vi "Create UA Client.vi"(8 "error in (no error)":errorcluster, 11 "OPCUA Setting In":T3) -> (0 "error out":errorcluster, 1 "Connected?":bool, 2 "NodeID Out":string, 3 "OPC UA client refnum out":T2)   [LabVIEW 2024, in "OPCUA.lvlib"]
uses:
  OPCUA.lvlib
  OPCUA Setting.ctl
  <vilib>/OPCUA/controls/OPC UA Client Refnum.ctl
  <vilib>/OPCUA/NI OPC UA Client.lvlib
panel:
  in  "security policy":T1
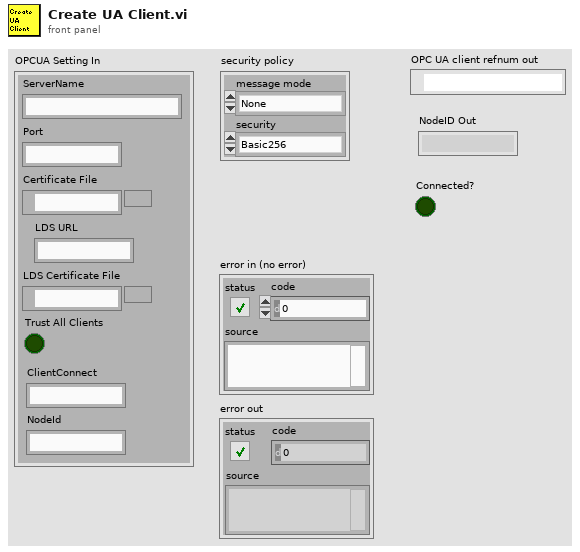
[diagram p1: front panel]
types:
  T1 = cluster{"message mode":enum16{"None", "Sign", "Sign and Encrypt"}, "security":enum16{"Basic256", "Basic128Rsa15"}}
  T2 = typedef "OPC UA Client Refnum.ctl" = refnum<k21>
  T3 = typedef "OPCUA.lvlib/OPCUA Setting.ctl" = cluster{"ServerName":string, "Port":string, "Certificate File":path, "LDS URL":string, "LDS Certificate File":path, "Trust All Clients":bool, "ClientConnect":string, "NodeId":string}
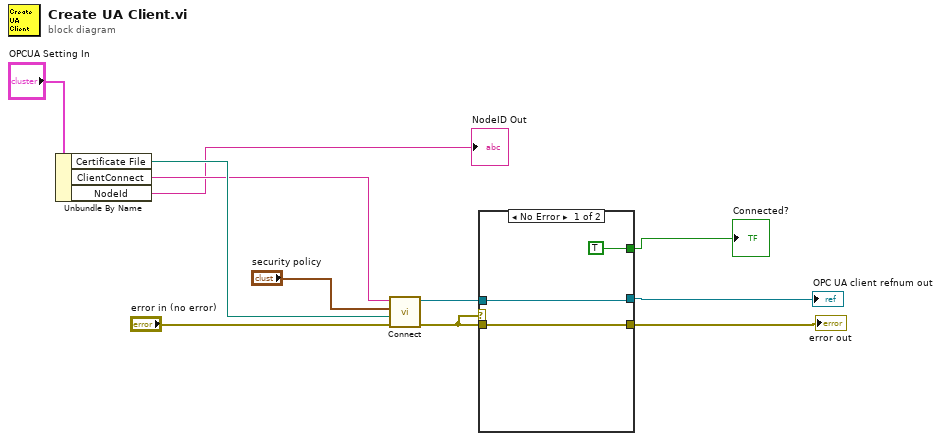
[diagram p0: block diagram]
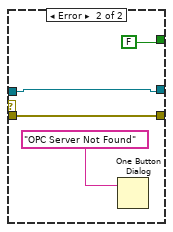
[diagram p2: hidden frame]
diagram:
  n1 = Unbundle By Name("OPCUA Setting In") -> ("Certificate File"=w9:path, "ClientConnect"=w7:string, "NodeId"=→"NodeID Out":string)
  n2 = call <vilib>:"Connect.vi"("error in (no error)"="error in (no error)", "client certificate file"=w9, "security policy"="security policy", "server endpoint URL"=w7) -> ("error out"=w1:errorcluster, "OPC UA client refnum out"=w5:T2)  [unwired: 5 in, 1 out]
  n3 = case shown="No Error" w1 {
    tunnel: w1 -> [w13 w16]
    tunnel: w5 -> [w14 w18]
    tunnel: [w14 w18] -> w4
    tunnel: [w13 w16] -> w3
    tunnel: [TRUE FALSE] -> w2
    frame No Error {
    }
    frame Error {
      n4 = One Button Dialog(message="OPC Server Not Found") -> ()  [unwired: 1 in, 1 out]
    }
  }
  "error out" <- w3
  "OPC UA client refnum out" <- w4
  "Connected?" <- w2
